vi "CRYSet Microphone Front Panel.vi"(11 "Vi Ref":refnum<vi>) -> ()   [LabVIEW 2013]
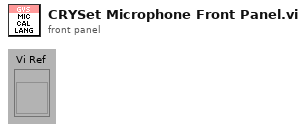
[diagram p1: front panel]
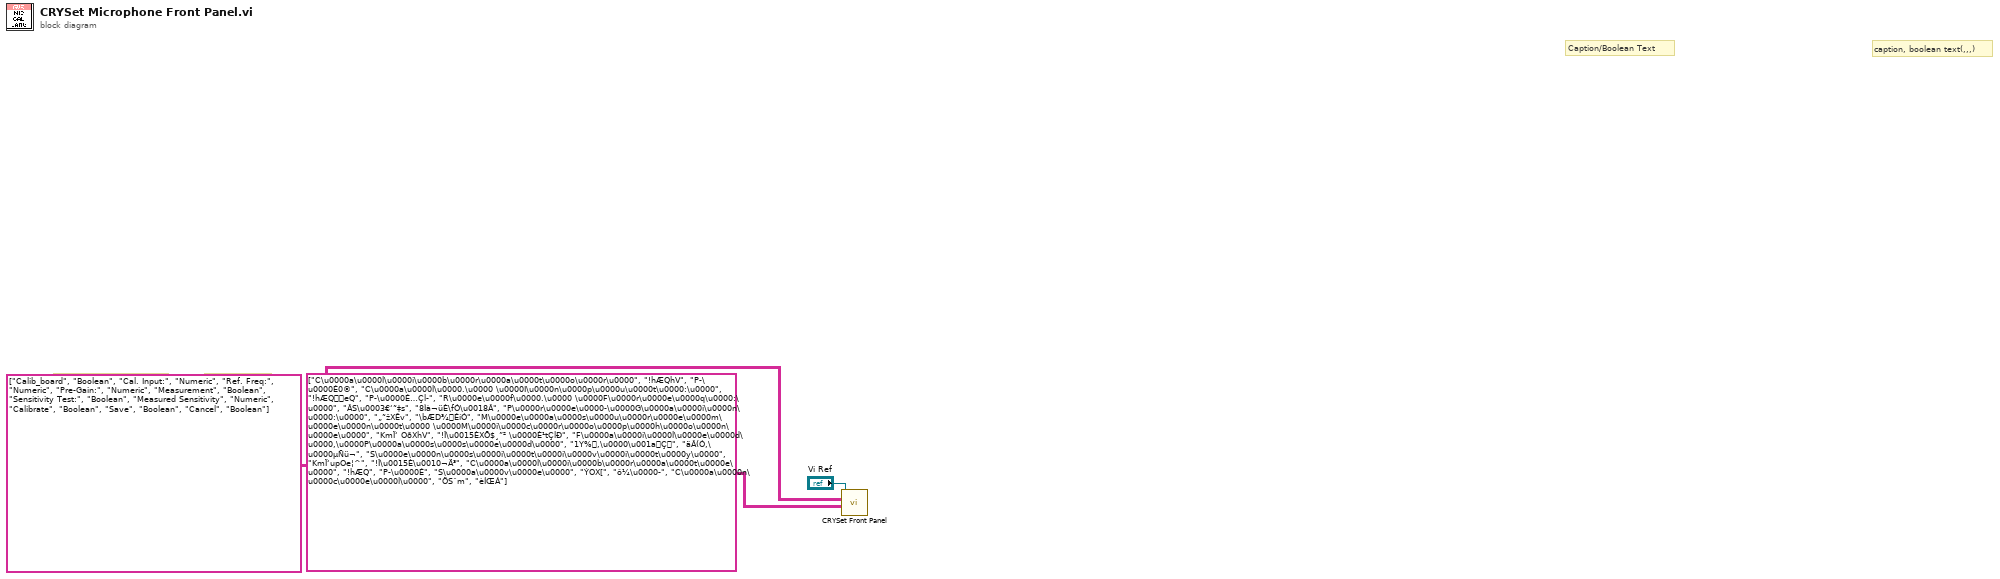
[diagram p0: block diagram]
diagram:
  # "Caption, Tab Page, Multilist Header, Button 4"
  # "Control Type"
  # "Control Name and Tab"
  # "caption, boolean text(,,,)"
  # "Caption/Boolean Text"
  n1 = call "CRYSet Front Panel.vi"("Caption(Boolean Text)"=string[][] [["C\u0000a\u0000l\u0000i\u0000b\u0000r\u0000a\u0000t\u0000o\u0000r\u0000", "!hÆQhV", "P­\u0000É0®"], ["C\u0000a\u0000l\u0000.\u0000 \u0000I\u0000n\u0000p\u0000u\u0000t\u0000:\u0000", "!hÆQeQ", "P­\u0000É…Çl­"], ["R\u0000e\u0000f\u0000.\u0000 \u0000F\u0000r\u0000e\u0000q\u0000:\u0000", "ÂS\u0003€‘˜‡s", "8Ìà¬üÈ\fÓ\u0018Â"], ["P\u0000r\u0000e\u0000-\u0000G\u0000a\u0000i\u0000n\u0000:\u0000", "„˜žXÊv", "\bÆD¾ÉíÓ"], ["M\u0000e\u0000a\u0000s\u0000u\u0000r\u0000e\u0000m\u0000e\u0000n\u0000t\u0000 \u0000M\u0000i\u0000c\u0000r\u0000o\u0000p\u0000h\u0000o\u0000n\u0000e\u0000", "KmÏ‘ OðXhV", "!Î\u0015ÈXÕ$¸”² \u0000È¹tÇlÐ"], ["F\u0000a\u0000i\u0000l\u0000e\u0000d\u0000,\u0000P\u0000a\u0000s\u0000s\u0000e\u0000d\u0000", "1Y%,\u0000\u001aÇ", "äÂ(Ó,\u0000µÑü¬"], ["S\u0000e\u0000n\u0000s\u0000i\u0000t\u0000i\u0000v\u0000i\u0000t\u0000y\u0000", "KmÏ‘upOe¦^", "!Î\u0015È\u0010¬Ä³"], ["C\u0000a\u0000l\u0000i\u0000b\u0000r\u0000a\u0000t\u0000e\u0000", "!hÆQ", "P­\u0000É"], ["S\u0000a\u0000v\u0000e\u0000", "ÝOX[", "ô¼\u0000­"], ["C\u0000a\u0000n\u0000c\u0000e\u0000l\u0000", "ÖSˆm", "èÍŒÁ"]], "Control ID and Type(Label Name, Type)"=string[][] [["Calib_board", "Boolean"], ["Cal. Input:", "Numeric"], ["Ref. Freq:", "Numeric"], ["Pre-Gain:", "Numeric"], ["Measurement", "Boolean"], ["Sensitivity Test:", "Boolean"], ["Measured Sensitivity", "Numeric"], ["Calibrate", "Boolean"], ["Save", "Boolean"], ["Cancel", "Boolean"]], "Vi Ref"="Vi Ref") -> ()  [unwired: 9 in]
